vi "Sort Complex Numbers (Real&Imag).vi"(10 "Order":enum16{"Ascending", "Descending"}(ring), 11 "Complex Numbers":cdb[](array[numeric]) format="%#.6g") -> (0 "error":i32, 2 "Sorted Index":i32[](array[numeric]), 3 "Sorted Complex Numbers":cdb[](array[numeric]) format="%#.6g")   [LabVIEW 2018, in "NI_AALPro.lvlib"]
doc: "Sorts an array of complex numbers in ascending or descending order with respect to their real and image parts."
uses:
  NI_AALPro.lvlib
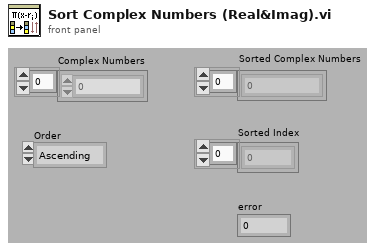
[diagram p1: front panel]
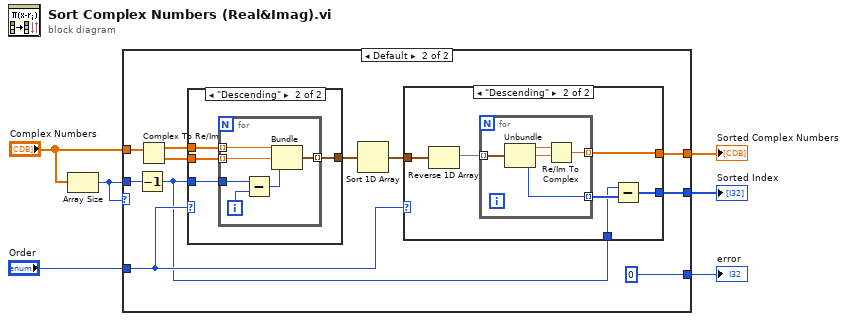
[diagram p0: block diagram]
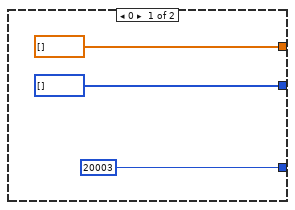
[diagram p2: hidden frame]
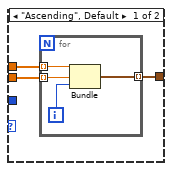
[diagram p3: hidden frame]
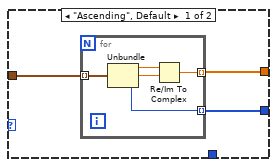
[diagram p4: hidden frame]
diagram:
  n1 = Array Size(array="Complex Numbers") -> (size(s)=w1:i32)
  n2 = case shown="Default" w1 {
    tunnel: "Complex Numbers" -> [_ w17]
    tunnel: [cdb[] [] ("CDB") w12] -> w6
    tunnel: [i32[] [] w11] -> w5
    tunnel: "Order" -> [_ w14]
    tunnel: [20003 ("empty array") 0] -> w2
    tunnel: w1 -> [_ w13]
    frame 0 {
    }
    frame Default {
      n3 = Decrement(x=w13) -> (x-1=w10:i32)
      n4 = Complex To Re/Im(x + iy=w17) -> (x=w19:dbl[], y=w18:dbl[])
      n5 = case shown="\"Descending\"" w14 {
        tunnel: [w23 w31] -> w20
        tunnel: w19 -> [w22 w30]
        tunnel: w18 -> [w21 w29]
        tunnel: w10 -> [_ w28]
        frame "Ascending", Default {
          n6 = for {
            tunnel: w22 -> [w27] mode=indexing
            tunnel: w21 -> [w25] mode=indexing
            tunnel: [w26] -> w23 mode=indexing
            i -> [w24]
            n7 = Bundle("Numeric"=w27, "Numeric"=w25, w24) -> (w26:cluster{"Numeric":dbl, "Numeric":dbl, i32})  [unwired: 1 in]
          }
        }
        frame "Descending" {
          n8 = for {
            tunnel: w30 -> [w37] mode=indexing
            tunnel: w29 -> [w35] mode=indexing
            tunnel: [w36] -> w31 mode=indexing
            tunnel: w28 -> [w33]
            i -> [w34]
            n9 = Subtract(x=w33, y=w34) -> (x-y=w32:i32)
            n10 = Bundle("Numeric"=w37, "Numeric"=w35, w32) -> (w36:cluster{"Numeric":dbl, "Numeric":dbl, i32})  [unwired: 1 in]
          }
        }
      }
      n11 = Sort 1D Array(array=w20) -> (sorted array=w16:cluster{"Numeric":dbl, "Numeric":dbl, i32}[])
      n12 = case shown="\"Descending\"" w14 {
        tunnel: w16 -> [w40 w51]
        tunnel: [w39 w46] -> w12
        tunnel: [w38 w47] -> w11
        tunnel: w10 -> [_ w48]
        frame "Ascending", Default {
          n13 = for {
            tunnel: w40 -> [w45] mode=indexing
            tunnel: [w42] -> w39 mode=indexing
            tunnel: [w41] -> w38 mode=indexing
            n14 = Unbundle(w45) -> ("Numeric"=w44:dbl, "Numeric"=w43:dbl, w41:i32)
            n15 = Re/Im To Complex(1:w43, 2:w44) -> (0:w42:cdb)
          }
        }
        frame "Descending" {
          n16 = Reverse 1D Array(array=w51) -> (reversed array=w50:cluster{"Numeric":dbl, "Numeric":dbl, i32}[])
          n17 = for {
            tunnel: w50 -> [w56] mode=indexing
            tunnel: [w53] -> w46 mode=indexing
            tunnel: [w52] -> w49 mode=indexing
            n18 = Unbundle(w56) -> ("Numeric"=w55:dbl, "Numeric"=w54:dbl, w52:i32)
            n19 = Re/Im To Complex(1:w54, 2:w55) -> (0:w53:cdb)
          }
          n20 = Subtract(x=w48, y=w49) -> (x-y=w47:i32[])
        }
      }
    }
  }
  "Sorted Complex Numbers" <- w6
  "Sorted Index" <- w5
  "error" <- w2
